vi "4ChannelAMCS-TwoChannel-Spuler_modified_13Nov1014.vi"() -> ()   [LabVIEW 2012]
uses:
  <vilib>/Analysis/baseanly.llb/Mean (DBL).vi
  Micropulse DIAL Labview/Scalar_Data_2.vi
  Micropulse DIAL Labview/Scalar_Data.vi
  AmcsUsb.dll
  <vilib>/Analysis/NI_AALBase.lvlib
panel:
  in  "length":i32=20
  in  "index":i32=200
  out "Total Counts 2":u16(graph)
  out "Waveform Graph 4":dbl[](graph)
  out "Waveform Graph 3":u16[](graph)
  out "return type":i32
  out "Waveform Graph 2":u16[](graph)=[19418, 38934, 12301, 4645, 4405, 4245, 4480, 4941, 5330, 5662, 6017, 6279, 6772, 6946, 6847, 6918, 6816, 6658, 6346, 6263, 6175, 5851, 5853, 5602, 5484, 5140, 5097, 4863, 4937, 4821, 4700, 4648, 4654, 4426, 4593, 4346, 4428, 4371, 4278, 4317, 4250, 4287, 4226, 4226, 4159, 4143, 4087, 4094, 4161, 4142, 4080, 4051, 4046, 4024, 4190, 4137, 3972, 4044, 4126, 4070, 4062, 4023, 3942, 4059, 4031, 3994, 3958, 4004, 3984, 3927, 4039, 4040, 4005, 4001, 3969, 3908, 3992, 3941, 3891, 4073, 3995, 4052, 3870, 3790, 3978, 4017, 4000, 4023, 3913, 4012, 3957, 4090, 3938, 3987, 3880, 4036, 3915, 3925, 3942, 3791, 3950, 3912, 4131, 4012, 4013, 4002, 4015, 3857, 4025, 3944, 3937, 3916, 4054, 3973, 3993, 3950, 3901, 3938, 3949, 4051, 3853, 3871, 3946, 3921, 3969, 3918, 3947, 3846, 4035, 3926, 3974, 3915, 4000, 3927, 3953, 3968, 4030, 3975, 3964, 3963, 3946, 3916, 3897, 4015, 3971, 3931, 3961, 4036, 3989, 4016, 4048, 3867, 4016, 3906, 4141, 4028, 3779, 3972, 4001, 3865, 3844, 4073, 3865, 3942, 4067, 4002, 3964, 3970, 3768, 3973, 4022, 3812, 3853, 3897, 3973, 3950, 3941, 3890, 4046, 3783, 3935, 3893, 4005, 3916, 3872, 4068, 3916, 3850, 4030, 4033, 3884, 3920, 4043, 3993, 3944, 3971, 3952, 4008, 3914, 3920, 3939, 3991, 3991, 3990, 3973, 3945, 3945, 3945, 4025, 4099, 3953, 3889, 3992, 3959, 3967, 3881, 3903, 3895, 4034, 4045]
  out "Total Counts":u16(graph)=2024
  in  "stop":bool
  out "Waveform Graph":dbl[](graph)=[15449.95, 34965.95, 8332.95, 676.9499999999998, 436.9499999999998, 276.9499999999998, 511.9499999999998, 972.9499999999998, 1361.9499999999998, 1693.9499999999998, 2048.95, 2310.95, 2803.95, 2977.95, 2878.95, 2949.95, 2847.95, 2689.95, 2377.95, 2294.95, 2206.95, 1882.9499999999998, 1884.9499999999998, 1633.9499999999998, 1515.9499999999998, 1171.9499999999998, 1128.9499999999998, 894.9499999999998, 968.9499999999998, 852.9499999999998, 731.9499999999998, 679.9499999999998, 685.9499999999998, 457.9499999999998, 624.9499999999998, 377.9499999999998, 459.9499999999998, 402.9499999999998, 309.9499999999998, 348.9499999999998, 281.9499999999998, 318.9499999999998, 257.9499999999998, 257.9499999999998, 190.94999999999982, 174.94999999999982, 118.94999999999982, 125.94999999999982, 192.94999999999982, 173.94999999999982, 111.94999999999982, 82.94999999999982, 77.94999999999982, 55.94999999999982, 221.94999999999982, 168.94999999999982, 3.949999999999818, 75.94999999999982, 157.94999999999982, 101.94999999999982, 93.94999999999982, 54.94999999999982, -26.050000000000182, 90.94999999999982, 62.94999999999982, 25.949999999999818, -10.050000000000182, 35.94999999999982, 15.949999999999818, -41.05000000000018, 70.94999999999982, 71.94999999999982, 36.94999999999982, 32.94999999999982, 0.9499999999998181, -60.05000000000018, 23.949999999999818, -27.050000000000182, -77.05000000000018, 104.94999999999982, 26.949999999999818, 83.94999999999982, -98.05000000000018, -178.05000000000018, 9.949999999999818, 48.94999999999982, 31.949999999999818, 54.94999999999982, -55.05000000000018, 43.94999999999982, -11.050000000000182, 121.94999999999982, -30.050000000000182, 18.949999999999818, -88.05000000000018, 67.94999999999982, -53.05000000000018, -43.05000000000018, -26.050000000000182, -177.05000000000018, -18.050000000000182, -56.05000000000018, 162.94999999999982, 43.94999999999982, 44.94999999999982, 33.94999999999982, 46.94999999999982, -111.05000000000018, 56.94999999999982, -24.050000000000182, -31.050000000000182, -52.05000000000018, 85.94999999999982, 4.949999999999818, 24.949999999999818, -18.050000000000182, -67.05000000000018, -30.050000000000182, -19.050000000000182, 82.94999999999982, -115.05000000000018, -97.05000000000018, -22.050000000000182, -47.05000000000018, 0.9499999999998181, -50.05000000000018, -21.050000000000182, -122.05000000000018, 66.94999999999982, -42.05000000000018, 5.949999999999818, -53.05000000000018, 31.949999999999818, -41.05000000000018, -15.050000000000182, -0.0500000000001819, 61.94999999999982, 6.949999999999818, -4.050000000000182, -5.050000000000182, -22.050000000000182, -52.05000000000018, -71.05000000000018, 46.94999999999982, 2.949999999999818, -37.05000000000018, -7.050000000000182, 67.94999999999982, 20.949999999999818, 47.94999999999982, 79.94999999999982, -101.05000000000018, 47.94999999999982, -62.05000000000018, 172.94999999999982, 59.94999999999982, -189.05000000000018, 3.949999999999818, 32.94999999999982, -103.05000000000018, -124.05000000000018, 104.94999999999982, -103.05000000000018, -26.050000000000182, 98.94999999999982, 33.94999999999982, -4.050000000000182, 1.949999999999818, -200.05000000000018, 4.949999999999818, 53.94999999999982, -156.05000000000018, -115.05000000000018, -71.05000000000018, 4.949999999999818, -18.050000000000182, -27.050000000000182, -78.05000000000018, 77.94999999999982, -185.05000000000018, -33.05000000000018, -75.05000000000018, 36.94999999999982, -52.05000000000018, -96.05000000000018, 99.94999999999982, -52.05000000000018, -118.05000000000018, 61.94999999999982, 64.94999999999982, -84.05000000000018, -48.05000000000018, 74.94999999999982, 24.949999999999818, -24.050000000000182, 2.949999999999818, -16.050000000000182, 39.94999999999982, -54.05000000000018, -48.05000000000018, -29.050000000000182, 22.949999999999818, 22.949999999999818, 21.949999999999818, 4.949999999999818, -23.050000000000182, -23.050000000000182, -23.050000000000182, 56.94999999999982, 130.94999999999982, -15.050000000000182, -79.05000000000018, 23.949999999999818, -9.050000000000182, -1.050000000000182, -87.05000000000018, -65.05000000000018, -73.05000000000018, 65.94999999999982, 76.94999999999982]
  out "Max. Rep. Rate (Hz)":dbl=9008.197459688316
  out "Data Collection Time per Column":dbl=1.1001
  in  "Channel":u16(ring) items=["Channel 1", "Channel 2", "Channel 3", "Channel 4"]
  out "MinSyncPulse\nPeriod":dbl=111.01 format="%.2f"
  in  "y units":u16(ring) items=["Bin #", "Sampling Time(µs)", "Range(m)"]
  in  "Time Resolution Per Bin(ns)":u16=500 min=5 max=1063 step=1
  in  "Number of Accumulates":u16=10000 min=1 max=32767 step=1
  in  "Number of Bins":u16=220 min=2 max=4095 step=1
  in  "Pulse A Polarity":enum16{"Low", "High"}(ring)=enum."High"
  in  "Sync Pulse Polarity":enum16{"Low", "High"}(ring)=enum."High"
  in  "Accumulation Delay(ns)":u16=10 min=10 max=1270 step=1
  in  "Pulse B Delay(ns)":u32=80 min=80 max=327600 step=1
  in  "Pulse A Delay(ns)":u32=80 min=80 max=327600
  in  "bins":u16=220 min=2 max=4095 step=1
  out "y offset":u16=10
  in  "ns scale":u16=500
  in  "Pulse B Polarity":enum16{"Low", "High"}(ring)=enum."High"
  out "Running?":bool
  out "Device ID":u32
  out "Open?":bool=TRUE
  # "Number of Accumulates"
  # "Time Resolution Per Bin(ns)"
  # "Accumulation Delay(ns)"
  # "Pulse A Delay(ns)"
  # "Far Field Returns (CH1)"
  # "Far Field Returns (CH1)"
  # "Pulse B Delay(ns)"
  # "Sync Pulse Polarity"
  # "Pulse A Polarity"
  # "Pulse B Polarity"
  # "Minimum Sync Pulse Period(µs)"
  # "Near Field Returns (CH2)"
  # "Near Field Returns (CH2)"
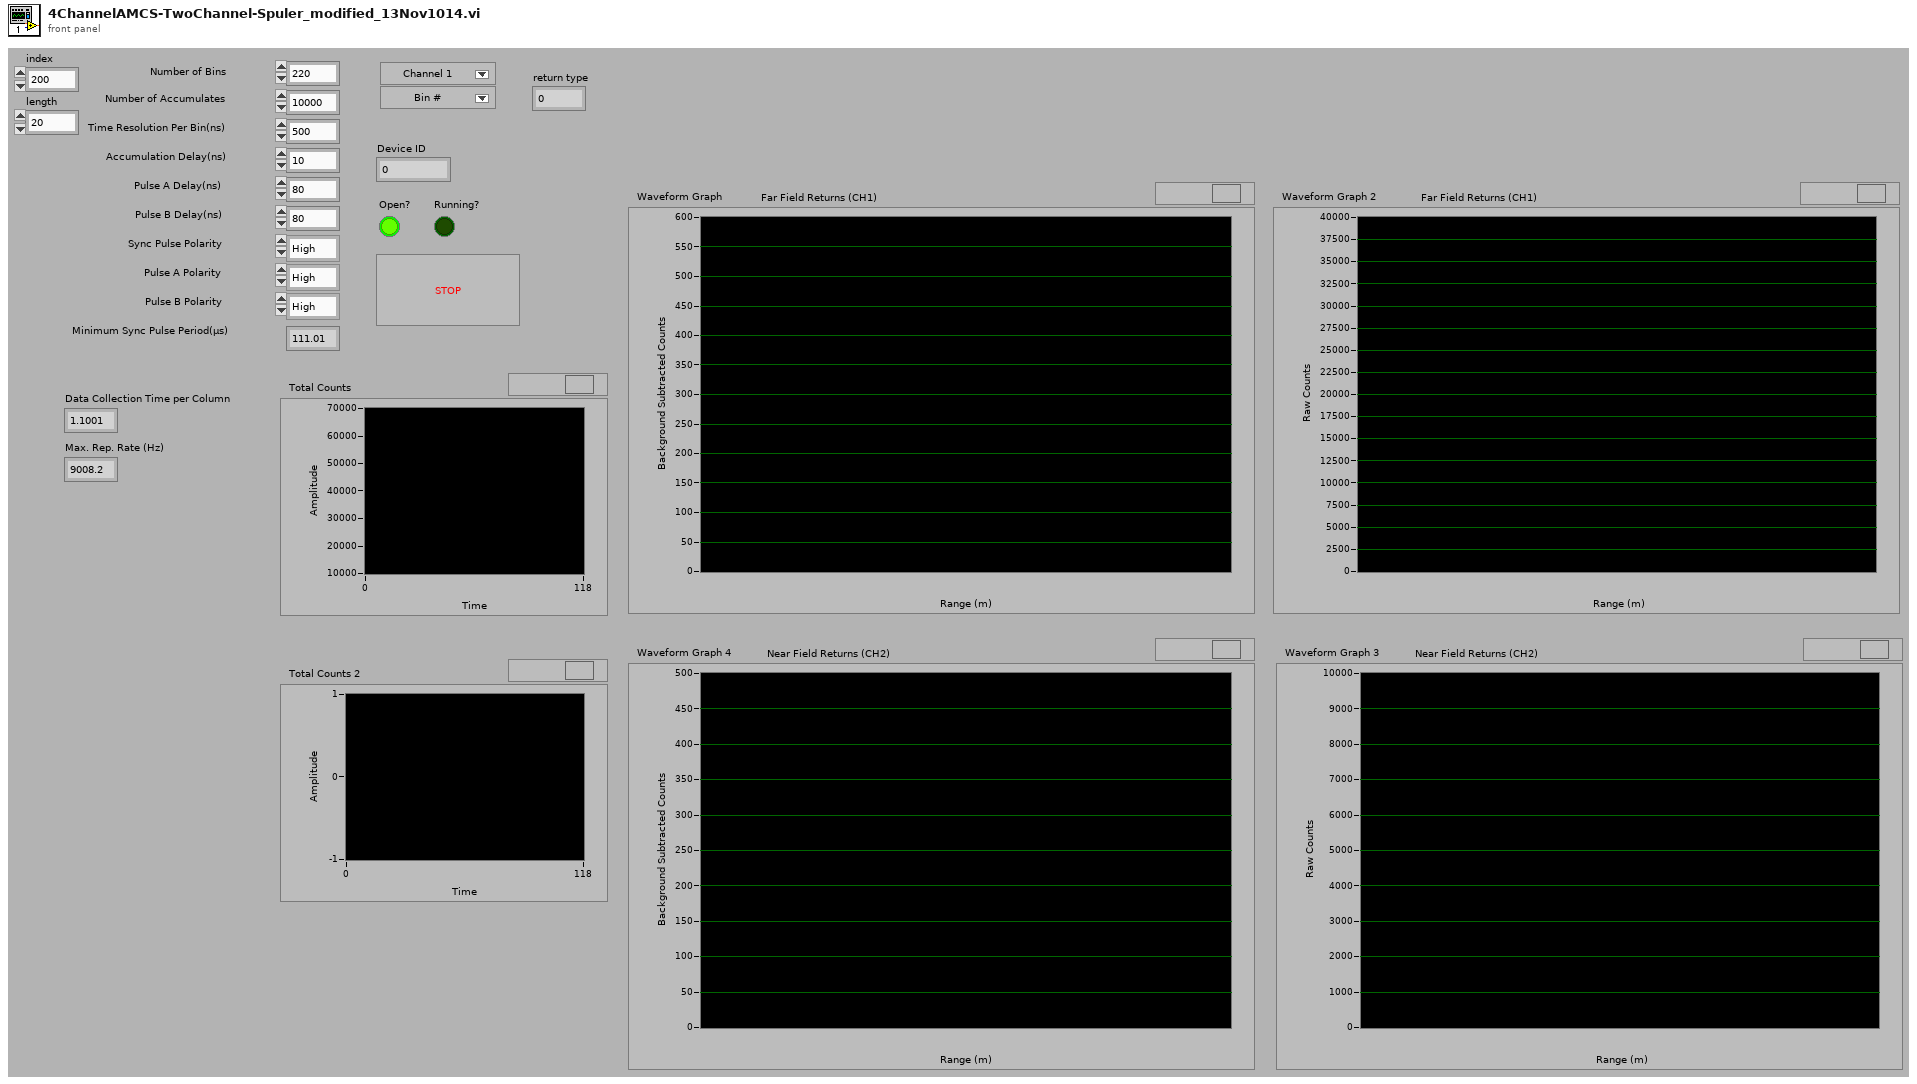
[diagram p1: front panel]
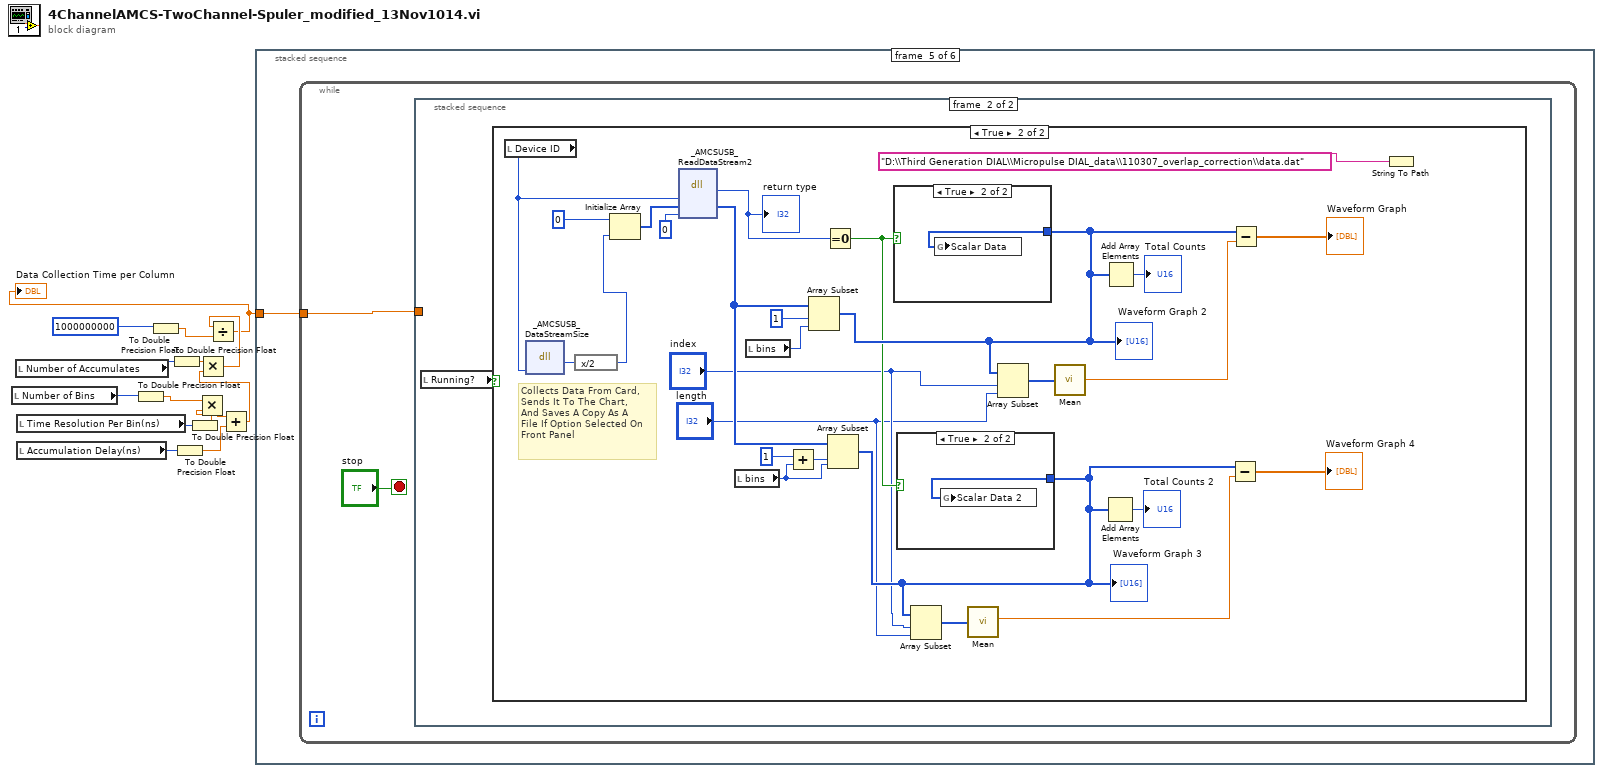
[diagram p0: block diagram]
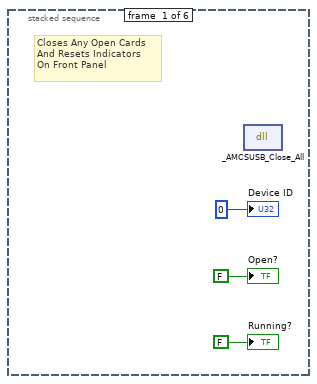
[diagram p2: hidden frame]
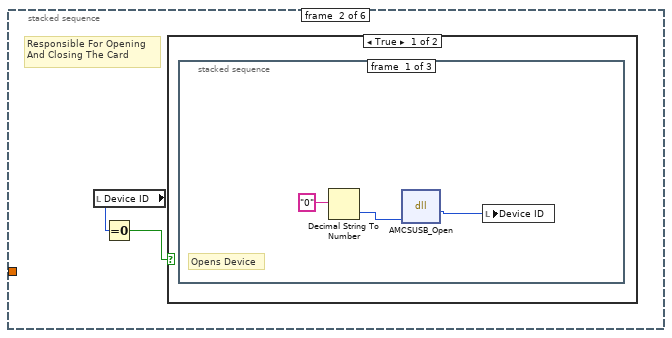
[diagram p3: hidden frame]
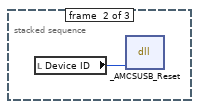
[diagram p4: hidden frame]
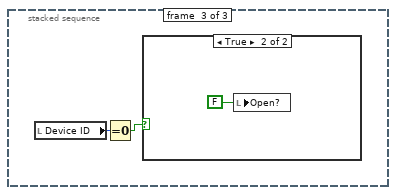
[diagram p5: hidden frame]
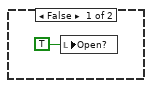
[diagram p6: hidden frame]
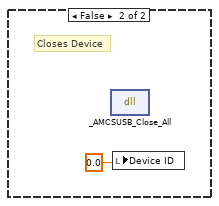
[diagram p7: hidden frame]
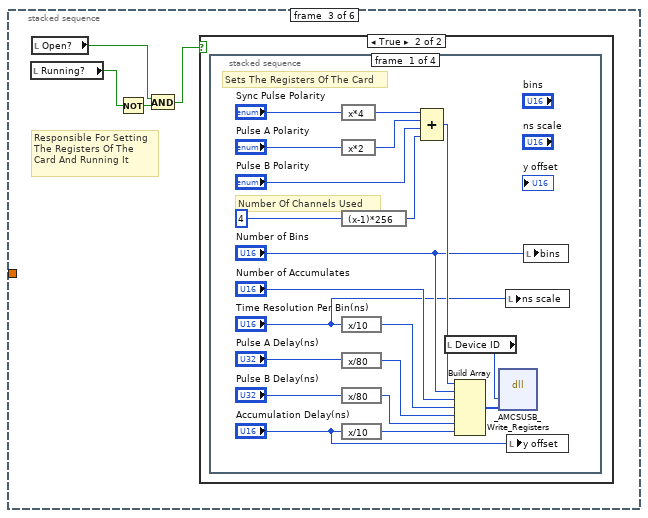
[diagram p8: hidden frame]
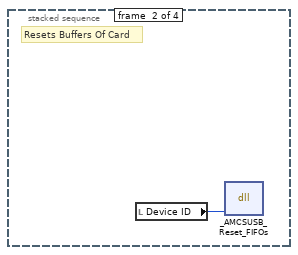
[diagram p10: hidden frame]
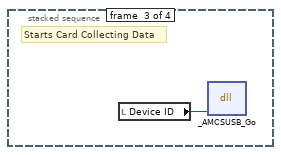
[diagram p11: hidden frame]
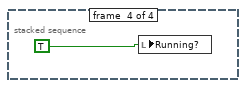
[diagram p12: hidden frame]
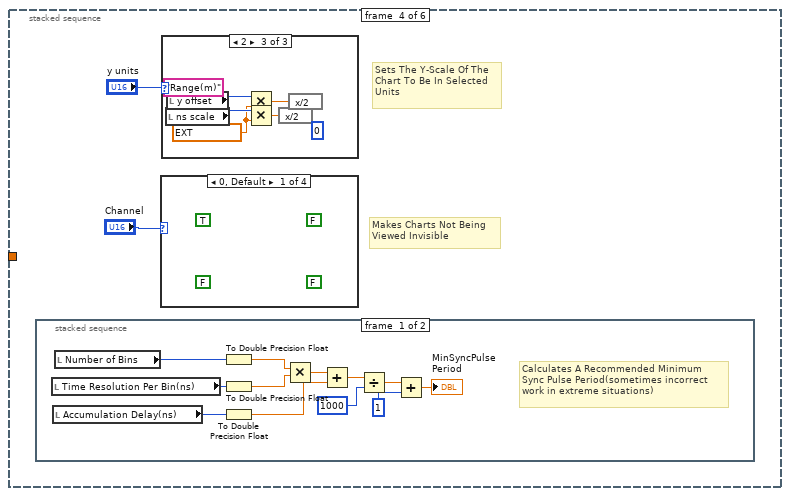
[diagram p13: hidden frame]
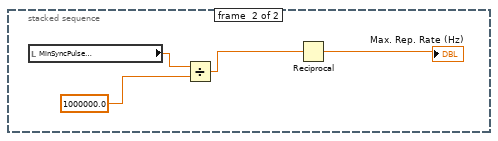
[diagram p14: hidden frame]
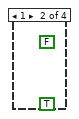
[diagram p15: hidden frame]
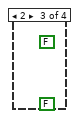
[diagram p16: hidden frame]
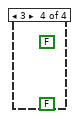
[diagram p17: hidden frame]
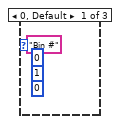
[diagram p18: hidden frame]
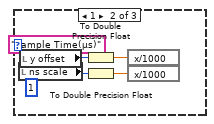
[diagram p19: hidden frame]
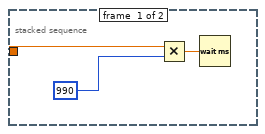
[diagram p20: hidden frame]
diagram:
  n1 = local read "Number of Bins"() -> (w5:u16)
  n2 = local read "Number of Accumulates"() -> (w10:u16)
  n3 = local read "Time Resolution Per Bin(ns)"() -> (w3:u16)
  n4 = local read "Accumulation Delay(ns)"() -> (w1:u16)
  n5 = To Double Precision Float(number=w5) -> (double precision float=w4:dbl)
  n6 = To Double Precision Float(number=1000000000) -> (double precision float=w7:dbl)
  n7 = To Double Precision Float(number=w10) -> (double precision float=w9:dbl)
  n8 = To Double Precision Float(number=w1) -> (double precision float=w2:dbl)
  n9 = To Double Precision Float(number=w3) -> (double precision float=w6:dbl)
  n10 = Multiply(x=w4, y=w6) -> (x*y=w14:dbl)
  n11 = Add(x=w14, y=w2) -> (x+y=w13:dbl)
  n12 = Multiply(x=w9, y=w13) -> (x*y=w12:dbl)
  n13 = Divide(x=w12, y=w7) -> (x/y=w11:dbl)
  "Data Collection Time per Column" <- w11
  n14 = stacked-sequence {
    tunnel: w11 -> [_ _ _ _ w83 _]
    frame #0 {
      # "Closes Any Open Cards\nAnd Resets Indicators\nOn Front Panel"
      n15 = dll-call lib="AmcsUsb.dll" fn="_AMCSUSB_Close_All" label="Close_All"() -> ()  [unwired: 4 in, 2 out]
      "Open?" <- FALSE ("Open?")
      "Device ID" <- u32 0 ("Device ID")
      "Running?" <- FALSE ("Running?")
    }
    frame #1 {
      # "Responsible For Opening\nAnd Closing The Card"
      n16 = local read "Device ID"() -> (w19:u32)
      n17 = Equal To 0?(x=w19) -> (x = 0?=w18:bool)
      n18 = case shown="True" w18 {
        frame True {
          # "Opens Device"
          n19 = stacked-sequence {
            frame #0 {
              n20 = Decimal String To Number(string="0" ("Device Number")) -> (number=w20:i32)  [unwired: 2 in, 1 out]
              n21 = dll-call lib="AmcsUsb.dll" fn="AMCSUSB_Open"("devnum"=w20) -> ("return type"=w21:u32)  [unwired: 4 in, 2 out]
              n22 = local write "Device ID"(w21) -> ()
            }
            frame #1 {
              n23 = local read "Device ID"() -> (w23:u32)
              n24 = dll-call lib="AmcsUsb.dll" fn="_AMCSUSB_Reset" label="Reset"("handle"=w23) -> ()  [unwired: 5 in, 2 out]
            }
            frame #2 {
              n25 = local read "Device ID"() -> (w24:u32)
              n26 = Equal To 0?(x=w24) -> (x = 0?=w25:bool)
              n27 = case shown="True" w25 {
                frame False {
                  n28 = local write "Open?"(TRUE ("Open?")) -> ()
                }
                frame True {
                  n29 = local write "Open?"(FALSE ("Open?")) -> ()
                }
              }
            }
          }
        }
        frame False {
          # "Closes Device"
          n30 = dll-call lib="AmcsUsb.dll" fn="_AMCSUSB_Close_All" label="Close_All"() -> ()  [unwired: 4 in, 2 out]
          n31 = local write "Device ID"(0.0 ("Device ID")) -> ()
        }
      }
    }
    frame #2 {
      # "Responsible For Setting\nThe Registers Of The\nCard And Running It"
      n32 = local read "Running?"() -> (w31:bool)
      n33 = local read "Open?"() -> (w32:bool)
      n34 = Not(x=w31) -> (.not. x?=w30:bool)
      n35 = And(x=w32, y=w30) -> (x .and. y?=w29:bool)
      n36 = case shown="True" w29 {
        frame False {
        }
        frame True {
          n37 = stacked-sequence {
            frame #0 {
              # "Sets The Registers Of The Card"
              # "Number Of Channels Used"
              n38 = expression code="x*4"("Sync Pulse Polarity") -> (w44:enum16{"Low", "High"})
              n39 = expression code="x*2"("Pulse A Polarity") -> (w34:enum16{"Low", "High"})
              n40 = expression code="(x-1)*256"(u32 4 ("Number of Channels Used")) -> (w43:u32)
              n41 = expression code="x/10"("Time Resolution Per Bin(ns)") -> (w37:u16)
              n42 = expression code="x/80"("Pulse A Delay(ns)") -> (w50:u32)
              n43 = expression code="x/80"("Pulse B Delay(ns)") -> (w52:u32)
              n44 = expression code="x/10"("Accumulation Delay(ns)") -> (w51:u16)
              n45 = Compound Arithmetic op=unknown(w44, w34, "Pulse B Polarity", w43) -> (w49:u32)
              n46 = local read "Device ID"() -> (w40:u32)
              n47 = Build Array(w49, "Number of Bins", "Number of Accumulates", w37, w50, w52, w51) -> (w42:u32[])
              n48 = dll-call lib="AmcsUsb.dll" fn="_AMCSUSB_Write_Registers" label="Write_Registers"("handle"=w40, "registers"=w42) -> ()  [unwired: 6 in, 2 out]
              n49 = local write "ns scale"("Time Resolution Per Bin(ns)") -> ()
              n50 = local write "y offset"("Accumulation Delay(ns)") -> ()
              n51 = local write "bins"("Number of Bins") -> ()
            }
            frame #1 {
              # "Resets Buffers Of Card"
              n52 = local read "Device ID"() -> (w53:u32)
              n53 = dll-call lib="AmcsUsb.dll" fn="_AMCSUSB_Reset_FIFOs" label="Reset_FIFOs"("handle"=w53) -> ()  [unwired: 5 in, 2 out]
            }
            frame #2 {
              # "Starts Card Collecting Data"
              n54 = local read "Device ID"() -> (w54:u32)
              n55 = dll-call lib="AmcsUsb.dll" fn="_AMCSUSB_Go" label="Go"("handle"=w54) -> ()  [unwired: 5 in, 2 out]
            }
            frame #3 {
              n56 = local write "Running?"(TRUE) -> ()
            }
          }
        }
      }
    }
    frame #3 {
      # "Makes Charts Not Being\nViewed Invisible"
      # "Sets The Y-Scale Of The\nChart To Be In Selected\nUnits"
      n57 = stacked-sequence {
        frame #0 {
          # "Calculates A Recommended Minimum\nSync Pulse Period(sometimes incorrect\nwork in extreme situations)"
          n58 = local read "Time Resolution Per Bin(ns)"() -> (w63:u16)
          n59 = local read "Accumulation Delay(ns)"() -> (w65:u16)
          n60 = local read "Number of Bins"() -> (w64:u16)
          n61 = To Double Precision Float(number=w64) -> (double precision float=w66:dbl)
          n62 = To Double Precision Float(number=w63) -> (double precision float=w67:dbl)
          n63 = To Double Precision Float(number=w65) -> (double precision float=w68:dbl)
          n64 = Multiply(x=w66, y=w67) -> (x*y=w62:dbl)
          n65 = Add(x=w62, y=w68) -> (x+y=w60:dbl)
          n66 = Divide(x=w60, y=u16 1000) -> (x/y=w59:dbl)
          n67 = Add(x=w59, y=u32 1) -> (x+y=→"MinSyncPulse\nPeriod":dbl)
        }
        frame #1 {
          n68 = local read "MinSyncPulse\nPeriod"() -> (w71:dbl)
          n69 = Divide(x=w71, y=1000000.0) -> (x/y=w70:dbl)
          n70 = Reciprocal(x=w70) -> (1/x=→"Max. Rep. Rate (Hz)":dbl)
        }
      }
      n71 = case shown="0, Default" "Channel" {
        frame 0, Default {
          (unwired) FALSE ("Visible")
          (unwired) FALSE ("Visible")
          (unwired) FALSE ("Visible")
          (unwired) TRUE ("Visible")
        }
        frame 1 {
          (unwired) FALSE ("Visible")
          (unwired) FALSE ("Visible")
          (unwired) TRUE ("Visible")
          (unwired) FALSE ("Visible")
        }
        frame 2 {
          (unwired) TRUE ("Visible")
          (unwired) FALSE ("Visible")
          (unwired) FALSE ("Visible")
          (unwired) FALSE ("Visible")
        }
        frame 3 {
          (unwired) FALSE ("Visible")
          (unwired) TRUE ("Visible")
          (unwired) FALSE ("Visible")
          (unwired) FALSE ("Visible")
        }
      }
      n72 = case shown="2" "y units" {
        frame 0, Default {
          (unwired) u8 0 ("Y Scale.Format & Precision:Precision")
          (unwired) u16 1 ("Y Scale.Offset and Multiplier:Multiplier")
          (unwired) "Bin #" ("Y Scale.Name Label.Text")
          (unwired) u16 0 ("Y Scale.Offset and Multiplier:Offset")
        }
        frame 1 {
          (unwired) u8 1 ("Y Scale.Format & Precision:Precision")
          (unwired) "Sample Time(µs)" ("Y Scale.Name Label.Text")
          n73 = local read "ns scale"() -> (w76:u16)
          n74 = local read "y offset"() -> (w77:u16)
          n75 = To Double Precision Float(number=w77) -> (double precision float=w75:dbl)
          n76 = To Double Precision Float(number=w76) -> (double precision float=w74:dbl)
          n77 = expression code="x/1000"(w75) -> ()  [unwired: 1 out]
          n78 = expression code="x/1000"(w74) -> ()  [unwired: 1 out]
        }
        frame 2 {
          (unwired) u8 0 ("Y Scale.Format & Precision:Precision")
          w78 = ext 0.299792458 ("y")
          (unwired) "Range(m)" ("Y Scale.Name Label.Text")
          n79 = local read "ns scale"() -> (w82:u16)
          n80 = local read "y offset"() -> (w81:u16)
          n81 = Multiply(x=w81, y=w78) -> (x*y=w80:ext)
          n82 = Multiply(x=w82, y=w78) -> (x*y=w79:ext)
          n83 = expression code="x/2"(w79) -> ()  [unwired: 1 out]
          n84 = expression code="x/2"(w80) -> ()  [unwired: 1 out]
        }
      }
    }
    frame #4 {
      n85 = while {
        tunnel: w83 -> [w85]
        stop <- "stop" stop-if-true
        n86 = stacked-sequence {
          tunnel: w85 -> [w88 _]
          frame #0 {
            n87 = Multiply(x=w88, y=990) -> (x*y=w86:dbl)
            n88 = Wait (ms)(milliseconds to wait=w86) -> ()  [unwired: 1 out]
          }
          frame #1 {
            n89 = local read "Running?"() -> (w89:bool)
            n90 = case shown="True" w89 {
              frame False {
              }
              frame True {
                # "Collects Data From Card,\nSends It To The Chart,\nAnd Saves A Copy As A\nFile If Option Selected On\nFront Panel"
                n91 = local read "Device ID"() -> (w113:u32)
                n92 = dll-call lib="AmcsUsb.dll" fn="_AMCSUSB_DataStreamSize" label="DataStreamSize"("handle"=w113) -> ("return type"=w106:u16)  [unwired: 4 in, 2 out]
                n93 = expression code="x/2"(w106) -> (w104:u16)
                n94 = Initialize Array(u32 0 ("element"), w104) -> (w114:u32[])
                n95 = dll-call lib="AmcsUsb.dll" fn="_AMCSUSB_ReadDataStream2" label="ReadDataStream2"("handle"=w113, "buffer"=w114, "BytesReturned"=u32 0) -> ("return type"=w105:i32, "buffer"=w95:u16[])  [unwired: 5 in, 2 out]
                "return type" <- w105
                n96 = local read "bins"() -> (w92:u16)
                n97 = local read "bins"() -> (w111:u16)
                n98 = Add(x=u16 1, y=w92) -> (x+y=w93:u16)
                n99 = Array Subset(array=w95, index=1 ("dimension size"), length=w111) -> (w103:u16[])
                "Waveform Graph 2" <- w103
                n100 = Equal To 0?(x=w105) -> (x = 0?=w96:bool)
                n101 = Array Subset(array=w95, index=w93, length=w92) -> (w97:u16[])
                "Waveform Graph 3" <- w97
                n102 = case shown="True" w96 {
                  tunnel: w103 -> [_ w118]
                  frame False {
                  }
                  frame True {
                    n103 = global write "Scalar_Data.vi" "Scalar Data"(w118) -> ()
                  }
                }
                n104 = case shown="True" w96 {
                  tunnel: w97 -> [_ w117]
                  frame False {
                  }
                  frame True {
                    n105 = global write "Scalar_Data_2.vi" "Scalar Data 2"(w117) -> ()
                  }
                }
                n106 = Array Subset(array=w97, index="index", length="length") -> (w101:u16[])
                n107 = call-poly <vilib>:"Mean.vi"("X"=w101) -> ("mean"=w98:dbl)  [unwired: 1 out]
                n108 = Array Subset(array=w103, index="index", length="length") -> (w110:u16[])
                n109 = call-poly <vilib>:"Mean.vi"("X"=w110) -> ("mean"=w109:dbl)  [unwired: 1 out]
                n110 = Add Array Elements(numeric array=w97) -> (sum=→"Total Counts 2":u16)
                n111 = Add Array Elements(numeric array=w103) -> (sum=→"Total Counts":u16)
                n112 = Subtract(x=w97, y=w98) -> (x-y=→"Waveform Graph 4":dbl[])
                n113 = Subtract(x=w103, y=w109) -> (x-y=→"Waveform Graph":dbl[])
                n114 = String To Path(string="D:\\Third Generation DIAL\\Micropulse DIAL_data\\110307_overlap_correction\\data.dat") -> ()  [unwired: 1 out]
              }
            }
          }
        }
      }
    }
    frame #5 {
      # "Closes Any Open Cards\nAnd Resets Indicators\nOn Front Panel"
      n115 = local write "Running?"(FALSE ("Running?")) -> ()
      n116 = local write "Open?"(TRUE ("Open?")) -> ()
      n117 = local write "Device ID"(u32 0 ("Device ID")) -> ()
      n118 = dll-call lib="AmcsUsb.dll" fn="_AMCSUSB_Close_All" label="Close_All"() -> ()  [unwired: 4 in, 2 out]
    }
  }
